vi "LabJackT4_Global.vi"() -> ()   [LabVIEW 2019]
panel:
  out "LJT4_P_HR3":dbl format="%.1f"
  out "LJT4_T":dbl format="%.1f"
  out "LJT4_ST":u32(colorbox)
  out "LJT4_P":dbl format="%.1f"
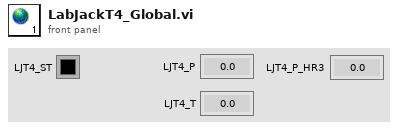
[diagram p1: front panel]
diagram:
